vi "HFRR ADV v02.vi"() -> ()   [LabVIEW 2025] (continued)
            n811 = call "CAMERA LIVE FEED FGV.vi"("Enum - Menu"=CAMERA_LIVE_FEED_ENUM."CAMERA MINIMIZE") -> ()  [unwired: 9 in, 2 out]
          }
        }
        n812 = local write "CAMERA ROI MAX TEMP"(TRUE ("CAMERA ROI MAX TEMP")) -> ()
        n813 = case shown="True" w1177 {
          selector: w1177 -> [_ w1183]
          frame False {
          }
          frame True {
            n814 = Not(x=w1183) -> (.not. x?=w1182:bool)
            n815 = local write "CAMERA ROI MIN TEMP"(w1182) -> ()
            n816 = call "IMAGE ANALYSIS.vi"("Enum"=POST_ANALYSIS_ENUM."MINIMIZE UI") -> ()  [unwired: 9 in, 2 out]
          }
        }
      }
    }
    n817 = local read "Auto Start Test"() -> (w928:bool)
    n818 = case shown="True" "sign in temp" {
      frame False {
      }
      frame True {
        w965 = 1 ("y")
        n819 = local read "USERNAME"() -> (w971:string)
        n820 = local read "USER ID"() -> (w968:string)
        n821 = call <vilib>:"Trim Whitespace.vi"("string"=w971) -> ("trimmed string"=w970:string)  [unwired: 1 in]
        n822 = call <vilib>:"Trim Whitespace.vi"("string"=w968) -> ("trimmed string"=w969:string)  [unwired: 1 in]
        n823 = String Length(string=w970) -> (length=w967:i32)
        n824 = String Length(string=w969) -> (length=w966:i32)
        n825 = Greater?(x=w967, y=w965) -> (0:w964:bool)
        n826 = Greater?(x=w966, y=w965) -> (0:w963:bool)
        n827 = And(x=w964, y=w963) -> (x .and. y?=w962:bool)
        n828 = case shown="True" w962 {
          frame False {
            n829 = property on="Sign In" class="Bool (strict)"("DisabledEnum"=T13."Disabled" ("Disabled")) -> ()  [unwired: 2 in, 2 out]
          }
          frame True {
            n830 = property on="Sign In" class="Bool (strict)"("DisabledEnum"=T13."Enabled" ("Disabled")) -> ()  [unwired: 2 in, 2 out]
          }
        }
      }
    }
    n831 = local read "Air Temperature"() -> (w945:bool)
    n832 = local read "Coefficient Of Friction"() -> (w946:bool)
    n833 = case shown="False" w928 {
      frame False {
        n834 = local read "Auto stop temp"() -> (w959:bool)
        n835 = case shown="True" w959 {
          frame False {
          }
          frame True {
            n836 = local write "Auto Start Temp"(FALSE ("Auto Start Temp")) -> ()
          }
        }
      }
      frame True {
        "Auto stop temp" <- TRUE ("Auto stop temp")
      }
    }
    n837 = local read "Humidity"() -> (w944:bool)
    n838 = case shown="\"HOME\"" w956 {
      frame "HOME" {
        n839 = local write "main tab sub"(enum32{"Page 1", "Page 2"}."Page 1" ("main tab sub")) -> ()
      }
      frame Default {
        n840 = local write "main tab sub"(enum32{"Page 1", "Page 2"}."Page 2" ("main tab sub")) -> ()
      }
    }
    n841 = case shown="True" w955 {
      selector: w955 -> [_ w1291]
      frame False {
      }
      frame True {
        n842 = Not(x=w1291) -> (.not. x?=w1290:bool)
        n843 = local write "Sign In"(w1290) -> ()
        n844 = local write "Main Dashboard Buttons"(T1."Test Setup" ("Main Dashboard Buttons")) -> ()
      }
    }
    n845 = case shown="\"Numeric Display\", Default" "Num/Graph" {
      frame "Numeric Display", Default {
        n846 = property on="Single/Multiple" class="RadioBtnsControl (strict)"("Visible"=FALSE) -> ()  [unwired: 2 in, 2 out]
        n847 = property on="Single - Graph" class="Ring (strict)"("Visible"=FALSE) -> ()  [unwired: 2 in, 2 out]
        n848 = local write "Main Tab Display"(T4."Dashboard 1" ("Main Tab Display")) -> ()
      }
      frame "Graph Display" {
        n849 = property on="Single/Multiple" class="RadioBtnsControl (strict)"("Visible"=TRUE) -> ()  [unwired: 2 in, 2 out]
        n850 = case shown="\"Multiple\"" "Single/Multiple" {
          frame "Single ", Default {
            n851 = property on="Single - Graph" class="Ring (strict)"("Visible"=TRUE) -> ()  [unwired: 2 in, 2 out]
            n852 = local write "Main Tab Display"(T4."Dashboard 3" ("Main Tab Display")) -> ()
          }
          frame "Multiple" {
            n853 = property on="Single - Graph" class="Ring (strict)"("Visible"=FALSE) -> ()  [unwired: 2 in, 2 out]
            n854 = local write "Main Tab Display"(T4."Dashboard 2" ("Main Tab Display")) -> ()
          }
        }
      }
    }
    n855 = local read "Stroke"() -> (w943:bool)
    n856 = local read "USERNAME"() -> (w949:string)
    n857 = local read "USER ID"() -> (w948:string)
    n858 = case shown="True" w946 {
      selector: w946 -> [_ w1226]
      frame False {
      }
      frame True {
        n859 = Not(x=w1226) -> (.not. x?=w1225:bool)
        n860 = local write "Coefficient Of Friction"(w1225) -> ()
        n861 = local write "Tab Control 2"(T6."Coefficient Of Friction" ("Tab Control 2")) -> ()
      }
    }
    n862 = case shown="True" w945 {
      selector: w945 -> [_ w1223]
      frame False {
      }
      frame True {
        n863 = Not(x=w1223) -> (.not. x?=w1221:bool)
        n864 = local write "Air Temperature"(w1221) -> ()
        n865 = local write "Tab Control 2"(T6."Air Temperature" ("Tab Control 2")) -> ()
      }
    }
    n866 = local write "Operator ID"(w948) -> ()
    n867 = case shown="True" w943 {
      selector: w943 -> [_ w1217]
      frame False {
      }
      frame True {
        n868 = Not(x=w1217) -> (.not. x?=w1215:bool)
        n869 = local write "Stroke"(w1215) -> ()
        n870 = local write "Tab Control 2"(T6."Stroke" ("Tab Control 2")) -> ()
      }
    }
    n871 = local write "tested by"(w949) -> ()
    n872 = case shown="True" w944 {
      selector: w944 -> [_ w1220]
      frame False {
      }
      frame True {
        n873 = Not(x=w1220) -> (.not. x?=w1218:bool)
        n874 = local write "Humidity"(w1218) -> ()
        n875 = local write "Tab Control 2"(T6."Humidity" ("Tab Control 2")) -> ()
      }
    }
    n876 = case shown="\"Advance\"" "Main Dashboard Buttons" {
      tunnel: [T2."HOME" ("Main Tab") T2."Test Setup" ("Main Tab") T2."Acquire" ("Main Tab") T2."Adv Scar" ("Main Tab") T2."Adv Scar Report" ("Main Tab") T2."Compare Files" ("Main Tab") T2."About" ("Main Tab") T2."Advance" ("Main Tab")] -> w953
      frame "Home", Default {
      }
      frame "Test Setup" {
      }
      frame "Dashboard" {
      }
      frame "Imaging" {
      }
      frame "Report" {
      }
      frame "Analysis" {
      }
      frame "About" {
      }
      frame "Advance" {
      }
    }
    n877 = Wait (ms)(milliseconds to wait=u32 100) -> ()  [unwired: 1 out]
    n878 = local read "Main Tab Display"() -> (w947:T4)
    n879 = local write "Main Tab"(w953) -> ()
    n880 = case shown="\"Dashboard 3\"" w947 {
      frame "Dashboard 1", Default {
        n881 = property on="Reset Graph" class="Bool (strict)"("Visible"=FALSE) -> ()  [unwired: 2 in, 2 out]
      }
      frame "Dashboard 2" {
        n882 = property on="Reset Graph" class="Bool (strict)"("Visible"=TRUE) -> ()  [unwired: 2 in, 2 out]
      }
      frame "Dashboard 3" {
        n883 = property on="Reset Graph" class="Bool (strict)"("Visible"=TRUE) -> ()  [unwired: 2 in, 2 out]
      }
    }
    n884 = local read "SCAR MEASURMENT"() -> (w935:enum32{"Auto Scar", "Manual Scar"})
    n885 = local read "Humidity"() -> (w950:bool)
    n886 = local read "Cap Live Image"() -> (w932:bool)
    n887 = local read "Sample Temperature"() -> (w942:bool)
    n888 = local read "Air Temp vs Humidity"() -> (w940:bool)
    n889 = local read "Frequency"() -> (w941:bool)
    n890 = case shown="False" w950 {
      frame False {
        n891 = local write "Humidity On Command"(TRUE ("Humidity On Command")) -> ()
        n892 = case shown="True" "Humidity Off Command" {
          selector: "Humidity Off Command" -> [_ w1233]
          frame False {
          }
          frame True {
            n893 = stacked-sequence {
              frame #0 {
                n894 = local read "WriteHumidity"() -> (w1235:string[])
                n895 = Insert Into Array(array=w1235, new element="R;1" ("new element/subarray")) -> (w1236:string[])  [unwired: 1 in]
                n896 = local write "WriteHumidity"(w1236) -> ()
              }
              frame #1 {
                n897 = Wait (ms)(milliseconds to wait=u32 2000) -> ()  [unwired: 1 out]
              }
              frame #2 {
                n898 = local read "EVENT LOG"() -> (w1242:string)
                n899 = local read "WriteHumidity"() -> (w1239:string[])
                n900 = call "Event Log.vi"("Content"="Humidity Control Off" ("string"), "EVENT LOG"=w1242) -> ("EVENT LOG"=w1243:string)  [unwired: 8 in, 1 out]
                n901 = local write "EVENT LOG"(w1243) -> ()
                n902 = Insert Into Array(array=w1239, new element="R;1" ("new element/subarray")) -> (w1240:string[])  [unwired: 1 in]
                n903 = local write "WriteHumidity"(w1240) -> ()
              }
            }
            n904 = Not(x=w1233) -> (.not. x?=w1232:bool)
            n905 = local write "Humidity Off Command"(w1232) -> ()
          }
        }
      }
      frame True {
        n906 = local write "Humidity Off Command"(TRUE ("Humidity Off Command")) -> ()
        n907 = case shown="False" "Humidity On Command" {
          selector: "Humidity On Command" -> [_ w1247]
          frame False {
          }
          frame True {
            n908 = stacked-sequence {
              frame #0 {
                n909 = local read "Set Rh"() -> (w1253:dbl)
                n910 = Number To Fractional String(number=w1253, precision (6)=i16 2) -> (F-format string=w1254:string)  [unwired: 2 in]
                n911 = local read "WriteHumidity"() -> (w1251:string[])
                n912 = Concatenate Strings("M;" ("new element/subarray"), w1254) -> (w1252:string)
                n913 = Insert Into Array(array=w1251, new element=w1252) -> (w1250:string[])  [unwired: 1 in]
                n914 = local write "WriteHumidity"(w1250) -> ()
              }
              frame #1 {
                n915 = Wait (ms)(milliseconds to wait=u32 1500) -> ()  [unwired: 1 out]
              }
              frame #2 {
                (unwired) "% RH" ("string")
                (unwired) i16 2 ("precision (6)")
                (unwired) "M;" ("new element/subarray")
                n916 = local read "Set Rh"() -> (w1261:dbl)
                n917 = Number To Fractional String(number=w1261, precision (6)=i16 2) -> (F-format string=w1258:string)  [unwired: 2 in]
                n918 = local read "WriteHumidity"() -> (w1263:string[])
                n919 = Concatenate Strings("M;" ("new element/subarray"), w1258) -> (w1262:string)
                n920 = Concatenate Strings("Humidity Set to : " ("string"), w1258, "% RH" ("string")) -> (w1256:string)
                n921 = Insert Into Array(array=w1263, new element=w1262) -> (w1264:string[])  [unwired: 1 in]
                n922 = disable-structure shown="Enabled" {
                  frame Enabled {
                    n923 = local read "EVENT LOG"() -> (w1267:string)
                    n924 = call "Event Log.vi"("Content"="Humidity Control On", "EVENT LOG"=w1267) -> ("EVENT LOG"=w1268:string)  [unwired: 8 in, 1 out]
                    n925 = local write "EVENT LOG"(w1268) -> ()
                  }
                  frame Disabled {
                  }
                }
                n926 = disable-structure shown="Enabled" {
                  disable-tunnel: w1256 -> [_ _]
                  frame Enabled {
                    n927 = local read "EVENT LOG"() -> (w1270:string)
                    n928 = call "Event Log.vi"("Content"="Humidity Control On", "EVENT LOG"=w1270) -> ("EVENT LOG"=w1271:string)  [unwired: 8 in, 1 out]
                    n929 = local write "EVENT LOG"(w1271) -> ()
                  }
                  frame Disabled {
                  }
                }
                n930 = local write "WriteHumidity"(w1264) -> ()
              }
            }
            n931 = Not(x=w1247) -> (.not. x?=w1246:bool)
            n932 = local write "Humidity On Command"(w1246) -> ()
          }
        }
      }
    }
    n933 = Equal?(x=w935, y=enum32{"Auto Scar", "Manual Scar"}."Auto Scar" ("SCAR MEASURMENT")) -> (x = y?=w931:bool)
    n934 = local read "TEST STANDARD"() -> (w938:T3)
    n935 = And(x=w932, y=w931) -> (x .and. y?=w933:bool)
    n936 = case shown="True" w933 {
      selector: w933 -> [_ w1032]
      tunnel: errorcluster {"status"=FALSE, "code"=0, "source"=""} ("error in (no error) 3") -> [_ w1033]
      frame False {
      }
      frame True {
        n937 = stacked-sequence {
          tunnel: w1033 -> [_ _ _ _ _ _ _ w1081]
          tunnel: w1032 -> [_ _ _ _ _ w1062 _ _]
          frame #0 {
            n938 = call "CAMERA LIVE FEED FGV.vi"("Enum - Menu"=CAMERA_LIVE_FEED_ENUM."CAMERA MINIMIZE") -> ()  [unwired: 9 in, 2 out]
          }
          frame #1 {
            n939 = property on="Auto Scar Check  2" class="Clust (strict)"("Visible"=TRUE) -> ()  [unwired: 2 in, 2 out]
          }
          frame #2 {
            n940 = String To Path(string="C:\\LAB-IQ\\Image Calibrate v01.dcf") -> (path=w1038:path)
            n941 = Open/Create/Replace File ("Open File")(file path (use dialog)=w1038) -> (refnum out=w1039:refnum<file>)  [unwired: 5 in, 2 out]
            n942 = for {
              N: 4 -> [_]
              tunnel: w1039 -> [w1045]
              i -> [w1041]
              n943 = Read from Text File ("Read File")(file (use dialog)=w1045) -> (text=w1046:string)  [unwired: 3 in, 3 out]
              n944 = String Subset(string=w1046, offset (0)=6, length (rest)=10 ("length (rest)")) -> (substring=w1042:string)
              n945 = Fract/Exp String To Number(string=w1042) -> (number=w1040:dbl)  [unwired: 3 in, 1 out]
              n946 = case shown="0" w1041 {
                tunnel: w1040 -> [w1047 w1048 _ w1049 _]
                frame 0 {
                  "5x Gain" <- w1047
                }
                frame 1 {
                  "10x Gain" <- w1048
                }
                frame 2 {
                }
                frame 3 {
                  "100x gain" <- w1049
                }
                frame 4, Default {
                }
              }
            }
          }
          frame #3 {
            n947 = local read "FILE 3"() -> (w1055:string)
            n948 = call <vilib>:"Trim Whitespace.vi"("string"="C:\\LAB-IQ\\images\\") -> ("trimmed string"=w1057:string)  [unwired: 1 in]
            n949 = String To Path(string=w1057) -> (path=w1056:path)
            n950 = Concatenate Strings(w1055, ".png" ("string")) -> (w1054:string)
            n951 = Build Path(base path=w1056, name or relative path=w1054) -> (appended path=w1052:path)
            "Image path" <- w1052
            n952 = Path To String(path=w1052) -> (string=w1051:string)
            n953 = call "CAMERA LIVE FEED FGV.vi"("Enum - Menu"=CAMERA_LIVE_FEED_ENUM."CAMERA SAVE", "Image Path"=w1051) -> ()  [unwired: 8 in, 2 out]
          }
          frame #4 {
            n954 = One Button Dialog(message="Image saved successfully") -> ()  [unwired: 1 in, 1 out]
          }
          frame #5 {
            n955 = local read "TEST STANDARD"() -> (w1061:T3)
            n956 = local read "Magnification len live scar"() -> (w1073:string)
            n957 = Not(x=w1062) -> (.not. x?=w1063:bool)
            n958 = local write "Cap Live Image"(w1063) -> ()
            n959 = case shown="\"ISO 12156\"" w1061 {
              tunnel: ["ASTM D6079" "ISO 12156"] -> w1060
              frame "ASTM D6079", Default {
              }
              frame "ISO 12156" {
              }
            }
            n960 = case shown="\"5x\", Default" w1073 {
              tunnel: [w1076 w1077] -> w1072
              frame "5x", Default {
                n961 = local read "5x Gain"() -> (w1076:dbl)
              }
              frame "10x" {
                # "5x"
                n962 = local read "10x Gain"() -> (w1077:dbl)
              }
            }
            n963 = local read "Image path"() -> (w1071:path)
            n964 = local read "FILE 3"() -> (w1064:string)
            n965 = call "EDGE DETCTION.vi"("GAIN VALUE"=w1072, "Image Path"=w1071) -> ("error out"=w1070:errorcluster, "return value"=w1069:cluster{string, string, dbl, dbl, dbl})  [unwired: 8 in]
            n966 = Bundle By Name(cluster=T18 {"File Name"="", "Test Method"="", "Operator"="", "Fuel Description"="", "Date and time"=""} ("Main Ref"), "File Name"=w1064, "Test Method"=w1060) -> (w1065:T18)
            n967 = call "duf file read.vi"("error in (no error)"=w1070, "Main Ref"=w1065) -> ("error out"=w1068:errorcluster, "Main Ref 2"=w1066:T18)  [unwired: 8 in]
            n968 = call "EDGE DETECTION REPORT.vi"("error in (no error)"=w1068, "return value 2"=w1069, "Main Ref"=w1066) -> ()  [unwired: 8 in, 1 out]
          }
          frame #6 {
            n969 = property on="Auto Scar Check  2" class="Clust (strict)"("Visible"=FALSE) -> ()  [unwired: 2 in, 2 out]
          }
          frame #7 {
            n970 = call "CAMERA LIVE FEED FGV.vi"("Enum - Menu"=CAMERA_LIVE_FEED_ENUM."CAMERA MINIMIZE", "error in (no error)"=w1081) -> ()  [unwired: 8 in, 2 out]
            n971 = local write "Main Dashboard Buttons"(T1."Home" ("Main Dashboard Buttons")) -> ()
            n972 = local write "Main Tab"(T2."HOME" ("Main Tab")) -> ()
          }
        }
      }
    }
    n973 = local read "Heater Button"() -> (w939:bool)
    n974 = case shown="True" w941 {
      selector: w941 -> [_ w1211]
      frame False {
      }
      frame True {
        n975 = Not(x=w1211) -> (.not. x?=w1209:bool)
        n976 = local write "Frequency"(w1209) -> ()
        n977 = local write "Tab Control 2"(T6."Frequency" ("Tab Control 2")) -> ()
      }
    }
    n978 = case shown="True" w940 {
      selector: w940 -> [_ w1208]
      frame False {
      }
      frame True {
        n979 = Not(x=w1208) -> (.not. x?=w1206:bool)
        n980 = local write "Air Temp vs Humidity"(w1206) -> ()
        n981 = local write "Tab Control 2"(T6."Air Temp vs Rh" ("Tab Control 2")) -> ()
      }
    }
    n982 = case shown="True" w942 {
      selector: w942 -> [_ w1214]
      frame False {
      }
      frame True {
        n983 = Not(x=w1214) -> (.not. x?=w1212:bool)
        n984 = local write "Sample Temperature"(w1212) -> ()
        n985 = local write "Tab Control 2"(T6."Sample Temperature" ("Tab Control 2")) -> ()
      }
    }
    n986 = case shown="\"Custom\"" w938 {
      frame "ASTM D6079", Default {
        w1187 = "ASTM D6079 TEST CONDITIONS" ("Standard 2")
        n987 = local write "Standard 2"(w1187) -> ()
        n988 = local write "Standard"(w1187) -> ()
      }
      frame "ISO 12156" {
        w1188 = "ISO 12156 TEST CONDITIONS" ("Standard 2")
        n989 = local write "Standard 2"(w1188) -> ()
        n990 = local write "Standard"(w1188) -> ()
      }
      frame "CEC F-096-A-06" {
        w1189 = "CEC F-096-A-06 TEST CONDITIONS" ("Standard 2")
        n991 = local write "Standard 2"(w1189) -> ()
        n992 = local write "Standard"(w1189) -> ()
      }
      frame "Custom" {
        w1190 = "CUSTOM TEST CONDITIONS" ("Standard 2")
        n993 = local write "Standard 2"(w1190) -> ()
        n994 = local write "Standard"(w1190) -> ()
      }
    }
    n995 = case shown="True" w939 {
      frame False {
        n996 = local write "Temperature On Command"(TRUE ("Temperature On Command")) -> ()
        n997 = case shown="True" "Temperature Off Command" {
          selector: "Temperature Off Command" -> [_ w1194]
          frame False {
          }
          frame True {
            n998 = Not(x=w1194) -> (.not. x?=w1193:bool)
            n999 = local read "EVENT LOG"() -> (w1197:string)
            n1000 = local write "Temperature Off Command"(w1193) -> ()
            n1001 = call "Event Log.vi"("Content"="Heater Off", "EVENT LOG"=w1197) -> ("EVENT LOG"=w1196:string)  [unwired: 8 in, 1 out]
            n1002 = local write "EVENT LOG"(w1196) -> ()
          }
        }
      }
      frame True {
        n1003 = local write "Temperature Off Command"(TRUE ("Temperature Off Command")) -> ()
        n1004 = case shown="True" "Temperature On Command" {
          selector: "Temperature On Command" -> [_ w1201]
          frame False {
          }
          frame True {
            n1005 = Not(x=w1201) -> (.not. x?=w1200:bool)
            n1006 = local write "Temperature On Command"(w1200) -> ()
            n1007 = disable-structure shown="Enabled" {
              disable-tunnel: "Heater On" -> [w1203 _]
              frame Enabled {
                n1008 = local read "EVENT LOG"() -> (w1204:string)
                n1009 = call "Event Log.vi"("Content"=w1203, "EVENT LOG"=w1204) -> ("EVENT LOG"=w1205:string)  [unwired: 8 in, 1 out]
                n1010 = local write "EVENT LOG"(w1205) -> ()
              }
              frame Disabled {
              }
            }
          }
        }
      }
    }
    n1011 = local read "Main Tab"() -> (w930:T2)
    n1012 = case shown="\"About\"" w930 {
      frame "HOME", Default {
        w976 = T13."Enabled" ("Disabled")
        n1013 = local read "Service Password enable"() -> (w975:bool)
        n1014 = property on="Imaging" class="Bool (strict)"("DisabledEnum"=w976) -> ()  [unwired: 2 in, 2 out]
        n1015 = property on="Dashboard" class="Bool (strict)"("DisabledEnum"=w976) -> ()  [unwired: 2 in, 2 out]
        n1016 = property on="Test Setup" class="Bool (strict)"("DisabledEnum"=w976) -> ()  [unwired: 2 in, 2 out]
        n1017 = property on="Analysis" class="Bool (strict)"("DisabledEnum"=w976) -> ()  [unwired: 2 in, 2 out]
        n1018 = property on="Home" class="Bool (strict)"("DisabledEnum"=w976) -> ()  [unwired: 2 in, 2 out]
        n1019 = property on="Report" class="Bool (strict)"("DisabledEnum"=w976) -> ()  [unwired: 2 in, 2 out]
        n1020 = property on="Main Dashboard Buttons" class="RadioBtnsControl (strict)"("DisabledEnum"=w976) -> ()  [unwired: 2 in, 2 out]
        n1021 = case shown="True" w975 {
          tunnel: [T13."Disabled" ("Disabled") T13."Enabled" ("Disabled")] -> w974
          frame False {
          }
          frame True {
          }
        }
        n1022 = property on="About" class="Bool (strict)"("DisabledEnum"=w974) -> ()  [unwired: 2 in, 2 out]
      }
      frame "Test Setup" {
        w981 = T13."Enabled" ("Disabled")
        n1023 = local read "Service Password enable"() -> (w980:bool)
        n1024 = property on="Dashboard" class="Bool (strict)"("DisabledEnum"=T13."Disabled" ("Disabled")) -> ()  [unwired: 2 in, 2 out]
        n1025 = property on="Imaging" class="Bool (strict)"("DisabledEnum"=w981) -> ()  [unwired: 2 in, 2 out]
        n1026 = property on="Analysis" class="Bool (strict)"("DisabledEnum"=w981) -> ()  [unwired: 2 in, 2 out]
        n1027 = property on="Home" class="Bool (strict)"("DisabledEnum"=w981) -> ()  [unwired: 2 in, 2 out]
        n1028 = property on="Report" class="Bool (strict)"("DisabledEnum"=w981) -> ()  [unwired: 2 in, 2 out]
        n1029 = property on="Test Setup" class="Bool (strict)"("DisabledEnum"=w981) -> ()  [unwired: 2 in, 2 out]
        n1030 = case shown="True" w980 {
          tunnel: [T13."Disabled" ("Disabled") T13."Enabled" ("Disabled")] -> w979
          frame False {
          }
          frame True {
          }
        }
        n1031 = property on="About" class="Bool (strict)"("DisabledEnum"=w979) -> ()  [unwired: 2 in, 2 out]
      }
      frame "Adv Scar" {
        w988 = T13."Enabled" ("Disabled")
        n1032 = property on="Dashboard" class="Bool (strict)"("DisabledEnum"=T13."Disabled" ("Disabled")) -> ()  [unwired: 2 in, 2 out]
        n1033 = property on="Imaging" class="Bool (strict)"("DisabledEnum"=w988) -> ()  [unwired: 2 in, 2 out]
        n1034 = property on="Analysis" class="Bool (strict)"("DisabledEnum"=w988) -> ()  [unwired: 2 in, 2 out]
        n1035 = property on="Home" class="Bool (strict)"("DisabledEnum"=w988) -> ()  [unwired: 2 in, 2 out]
        n1036 = property on="Report" class="Bool (strict)"("DisabledEnum"=w988) -> ()  [unwired: 2 in, 2 out]
        n1037 = property on="Test Setup" class="Bool (strict)"("DisabledEnum"=w988) -> ()  [unwired: 2 in, 2 out]
        n1038 = local read "Service Password enable"() -> (w986:bool)
        n1039 = case shown="True" w986 {
          tunnel: [T13."Disabled" ("Disabled") T13."Enabled" ("Disabled")] -> w985
          frame False {
          }
          frame True {
          }
        }
        n1040 = property on="About" class="Bool (strict)"("DisabledEnum"=w985) -> ()  [unwired: 2 in, 2 out]
      }
      frame "Adv Scar Report" {
        w993 = T13."Enabled" ("Disabled")
        n1041 = property on="Dashboard" class="Bool (strict)"("DisabledEnum"=T13."Disabled" ("Disabled")) -> ()  [unwired: 2 in, 2 out]
        n1042 = property on="Imaging" class="Bool (strict)"("DisabledEnum"=w993) -> ()  [unwired: 2 in, 2 out]
        n1043 = property on="Analysis" class="Bool (strict)"("DisabledEnum"=w993) -> ()  [unwired: 2 in, 2 out]
        n1044 = property on="Home" class="Bool (strict)"("DisabledEnum"=w993) -> ()  [unwired: 2 in, 2 out]
        n1045 = property on="Report" class="Bool (strict)"("DisabledEnum"=w993) -> ()  [unwired: 2 in, 2 out]
        n1046 = property on="Test Setup" class="Bool (strict)"("DisabledEnum"=w993) -> ()  [unwired: 2 in, 2 out]
        n1047 = local read "Service Password enable"() -> (w992:bool)
        n1048 = case shown="True" w992 {
          tunnel: [T13."Disabled" ("Disabled") T13."Enabled" ("Disabled")] -> w991
          frame False {
          }
          frame True {
          }
        }
        n1049 = property on="About" class="Bool (strict)"("DisabledEnum"=w991) -> ()  [unwired: 2 in, 2 out]
      }
      frame "Compare Files" {
        w999 = T13."Enabled" ("Disabled")
        n1050 = local read "Service Password enable"() -> (w998:bool)
        n1051 = property on="Dashboard" class="Bool (strict)"("DisabledEnum"=T13."Disabled" ("Disabled")) -> ()  [unwired: 2 in, 2 out]
        n1052 = property on="Imaging" class="Bool (strict)"("DisabledEnum"=w999) -> ()  [unwired: 2 in, 2 out]
        n1053 = property on="Analysis" class="Bool (strict)"("DisabledEnum"=w999) -> ()  [unwired: 2 in, 2 out]
        n1054 = property on="Home" class="Bool (strict)"("DisabledEnum"=w999) -> ()  [unwired: 2 in, 2 out]
        n1055 = property on="Report" class="Bool (strict)"("DisabledEnum"=w999) -> ()  [unwired: 2 in, 2 out]
        n1056 = property on="Test Setup" class="Bool (strict)"("DisabledEnum"=w999) -> ()  [unwired: 2 in, 2 out]
        n1057 = case shown="True" w998 {
          tunnel: [T13."Disabled" ("Disabled") T13."Enabled" ("Disabled")] -> w997
          frame False {
          }
          frame True {
          }
        }
        n1058 = property on="About" class="Bool (strict)"("DisabledEnum"=w997) -> ()  [unwired: 2 in, 2 out]
      }
      frame "Acquire" {
        n1059 = local read "Service Password enable"() -> (w1003:bool)
        n1060 = property on="Test Setup" class="Bool (strict)"("DisabledEnum"=T13."Disabled" ("Disabled")) -> ()  [unwired: 2 in, 2 out]
        n1061 = local read "Auto Start Test"() -> (w1005:bool)
        n1062 = local read "RUN"() -> (w1007:bool)
        n1063 = case shown="True" w1003 {
          tunnel: [T13."Disabled" ("Disabled") T13."Enabled" ("Disabled")] -> w1004
          frame False {
          }
          frame True {
          }
        }
        n1064 = Or(x=w1007, y=w1005) -> (x .or. y?=w1006:bool)
        n1065 = case shown="True" w1006 {
          tunnel: [T13."Enabled" ("Disabled") T13."Disabled" ("Disabled")] -> w1009
          frame False {
          }
          frame True {
          }
        }
        n1066 = property on="About" class="Bool (strict)"("DisabledEnum"=w1004) -> ()  [unwired: 2 in, 2 out]
        n1067 = property on="Imaging" class="Bool (strict)"("DisabledEnum"=w1009) -> ()  [unwired: 2 in, 2 out]
        n1068 = property on="Dashboard" class="Bool (strict)"("DisabledEnum"=w1009) -> ()  [unwired: 2 in, 2 out]
        n1069 = property on="Analysis" class="Bool (strict)"("DisabledEnum"=w1009) -> ()  [unwired: 2 in, 2 out]
        n1070 = property on="Home" class="Bool (strict)"("DisabledEnum"=w1009) -> ()  [unwired: 2 in, 2 out]
        n1071 = property on="Report" class="Bool (strict)"("DisabledEnum"=w1009) -> ()  [unwired: 2 in, 2 out]
      }
      frame "About" {
        n1072 = local read "FILE"() -> (w1022:string)
        n1073 = local read "TEST FILE NAM,E SAVED"() -> (w1015:bool)
        n1074 = call <vilib>:"Trim Whitespace.vi"("string"=w1022) -> ("trimmed string"=w1021:string)  [unwired: 1 in]
        n1075 = local read "Auto Start Test"() -> (w1025:bool)
        n1076 = String Length(string=w1021) -> (length=w1020:i32)
        n1077 = Greater?(x=w1020, y=1) -> (0:w1017:bool)
        n1078 = And(x=w1017, y=w1015) -> (x .and. y?=w1016:bool)
        n1079 = local read "RUN"() -> (w1027:bool)
        n1080 = case shown="True" w1016 {
          tunnel: [T13."Disabled" ("Disabled") T13."Enabled" ("Disabled")] -> w1018
          frame False {
          }
          frame True {
          }
        }
        n1081 = Or(x=w1027, y=w1025) -> (x .or. y?=w1026:bool)
        n1082 = property on="About" class="Bool (strict)"("DisabledEnum"=T13."Enabled" ("Disabled")) -> ()  [unwired: 2 in, 2 out]
        n1083 = case shown="False" w1026 {
          tunnel: [T13."Enabled" ("Disabled") T13."Disabled" ("Disabled")] -> w1024
          frame False {
          }
          frame True {
          }
        }
        n1084 = property on="Dashboard" class="Bool (strict)"("DisabledEnum"=w1018) -> ()  [unwired: 2 in, 2 out]
        n1085 = property on="Test Setup" class="Bool (strict)"("DisabledEnum"=T13."Disabled" ("Disabled")) -> ()  [unwired: 2 in, 2 out]
        n1086 = property on="Imaging" class="Bool (strict)"("DisabledEnum"=w1024) -> ()  [unwired: 2 in, 2 out]
        n1087 = property on="Analysis" class="Bool (strict)"("DisabledEnum"=w1024) -> ()  [unwired: 2 in, 2 out]
        n1088 = property on="Home" class="Bool (strict)"("DisabledEnum"=w1024) -> ()  [unwired: 2 in, 2 out]
        n1089 = property on="Report" class="Bool (strict)"("DisabledEnum"=w1024) -> ()  [unwired: 2 in, 2 out]
      }
    }
    n1090 = local read "Quit"() -> (w958:bool)
    "Single" <- "Single - Graph"
  }
  n1091 = disable-structure shown="Disabled" {
    disable-tunnel: [w1295 _] -> w39
    disable-tunnel: _ -> [w1294 _]
    frame Disabled {
      n1092 = while {
        tunnel: w1294 -> [_]
        tunnel: [w1296] -> w1295
        tunnel: [w1297] -> _
        i -> [w1297]
        stop <- w1296 stop-if-true
        w1313 = u16 10 items=["1.0"=10, "1.5"=15, "2.0"=20] ("stop bits (10: 1 bit)")
        n1093 = Wait (ms)(milliseconds to wait=u32 10) -> ()  [unwired: 1 out]
        n1094 = call-poly "VISA Configure Serial Port"("VISA resource name"=refnum<visa-resource-name> "ASRL1::INSTR" ("COM PORT"), "timeout (10sec)"=u32 10, "baud rate (9600)"=u32 57600, "data bits (8)"=u16 8, "stop bits (10: 1 bit)"=w1313) -> ("VISA resource name out"=w1299:refnum<visa-resource-name>, "error out"=w1308:errorcluster)  [unwired: 9 in]
        n1095 = VISA Read(VISA resource name=w1299, byte count=u32 2 ("byte count (0)")) -> (read buffer=w1307:string)  [unwired: 1 in, 3 out]
        n1096 = String Subset(string=w1307, offset (0)=0, length (rest)=2 ("length (rest)")) -> (substring=w1306:string)
        n1097 = Match Pattern(string=w1306, regular expression="<>") -> (offset past match=w1303:i32)  [unwired: 1 in, 3 out]
        n1098 = Greater Or Equal?(x=w1303, y=0) -> (x >= y?=w1298:bool)
        n1099 = case shown="True" w1298 {
          tunnel: w1299 -> [_ w1317]
          tunnel: w1308 -> [_ w1316]
          frame False {
          }
          frame True {
            n1100 = VISA Read(VISA resource name=w1317, byte count=u32 32 ("byte count (0)"), error in (no error)=w1316) -> (read buffer=w1315:string)  [unwired: 3 out]
            n1101 = String Subset(string=w1315, offset (0)=0, length (rest)=8 ("length (rest)")) -> (substring=w1319:string)
            n1102 = String Subset(string=w1315, offset (0)=8, length (rest)=8 ("length (rest)")) -> (substring=w1320:string)
            n1103 = Decimal String To Number(string=w1320) -> (number=w1327:i32)  [unwired: 2 in, 1 out]
            n1104 = Decimal String To Number(string=w1319) -> (number=w1323:i32)  [unwired: 2 in, 1 out]
            n1105 = Divide(x=w1327, y=10000) -> ()  [unwired: 1 out]
            n1106 = Divide(x=w1323, y=1000000) -> ()  [unwired: 1 out]
          }
        }
        n1107 = local read "Quit"() -> (w1296:bool)
      }
    }
    frame Enabled {
    }
  }
  n1108 = while {
    shift-right: [w1342] -> w52
    shift-left: _ -> [w1333]
    shift-right: [w1341] -> w51
    shift-left: errorcluster {"status"=TRUE, "code"=0, "source"="Init"} ("error IO") -> [w1335]
    tunnel: [w1330] -> w42
    tunnel: [w1340] -> _
    i -> [w1340]
    stop <- w1330 stop-if-true
    n1109 = local read "Port 1a"() -> (w1336:bool)
    n1110 = local read "Port 3"() -> (w1337:bool)
    n1111 = local read "Com Port 1"() -> (w1334:refnum<visa-resource-name>)
    n1112 = Or(x=w1337, y=w1336) -> (x .or. y?=w1339:bool)
    n1113 = Unbundle(w1335) -> ("status"=→"Port 3":bool)  [unwired: 2 out]
    n1114 = Not Equal?(x=w1334, y=w1333) -> (x != y?=w1331:bool)
    n1115 = case shown="True" w1339 {
      frame False {
        w1345 = FALSE ("Visible")
        n1116 = property on="Port 1a" class="Bool (strict)"("Visible"=w1345) -> ()  [unwired: 2 in, 2 out]
        n1117 = property on="Port 3" class="Bool (strict)"("Visible"=w1345) -> ()  [unwired: 2 in, 2 out]
      }
      frame True {
        w1346 = TRUE ("Visible")
        n1118 = property on="Port 1a" class="Bool (strict)"("Visible"=w1346) -> ()  [unwired: 2 in, 2 out]
        n1119 = property on="Port 3" class="Bool (strict)"("Visible"=w1346) -> ()  [unwired: 2 in, 2 out]
      }
    }
    n1120 = Wait (ms)(milliseconds to wait=u32 10) -> ()  [unwired: 1 out]
    n1121 = case shown="True" w1331 {
      tunnel: [w1343 errorcluster {"status"=TRUE, "code"=0, "source"="Init"} ("error out")] -> w1332
      tunnel: w1335 -> [w1343 _]
      frame False {
      }
      frame True {
      }
    }
    n1122 = case shown="No Error" w1332 {
      selector: w1332 -> [w1353 w1380]
      tunnel: [w1356 w1384] -> w1342
      tunnel: [w1355 w1378] -> w1341
      tunnel: w1333 -> [w1354 w1382]
      frame No Error {
        n1123 = property class="Instr"(reference=w1354, error in=w1353) -> (reference out=w1351:refnum<visa-resource-name>, error out=w1352:errorcluster, "Serial Settings:Number of Bytes at Serial Port"=w1347:u32)
        n1124 = Greater?(x=w1347, y=u32 5) -> (0:w1349:bool)
        n1125 = Not(x=w1349) -> (.not. x?=→"Port 1a":bool)
        n1126 = while {
          tunnel: [w1373] -> w1355
          tunnel: [w1372] -> w1356
          tunnel: w1352 -> [w1371]
          tunnel: w1351 -> [w1370]
          stop <- TRUE stop-if-true
          n1127 = property class="Instr" props=["Serial Settings:Number of Bytes at Serial Port"](reference=w1370, error in=w1371) -> (reference out=w1375:refnum<visa-resource-name>, error out=w1374:errorcluster)  [unwired: 1 out]
          n1128 = VISA Read(VISA resource name=w1375, byte count=u32 1000, error in (no error)=w1374) -> (VISA resource name out=w1372:refnum<visa-resource-name>, read buffer=w1357:string, error out=w1373:errorcluster)  [unwired: 1 out]
          "UNI READ" <- w1357
          n1129 = Spreadsheet String To Array(delimiter (Tab)=";", format string="", spreadsheet string=w1357, array type (2D Dbl)=dbl[] []) -> (array=w1367:dbl[])
          n1130 = Index Array(array=w1367) -> (element #1=→"LVDT MIN":dbl, element #2=→"LVDT MAX":dbl, element #3=→"LVDT Peak":dbl, element #4=→"pizo raw":dbl, element #5=→"Friction":dbl, element #6=→"cof 2":dbl)  [unwired: 6 in]
        }
      }
      frame Error {
        w1390 = u16 0 items=["None", "XON/XOFF", "RTS/CTS", "XON/XOFF & RTS/CTS", "DTR/DSR", "XON/XOFF & DTR/DSR"] ("flow control (0:none)  2")
        w1388 = u16 10 items=["1.0"=10, "1.5"=15, "2.0"=20] ("stop bits 2")
        w1386 = u16 0 items=["None", "Odd", "Even", "Mark", "Space"] ("parity 2")
        w1387 = u32 10000  # timeout (10sec)
        n1131 = VISA Close(VISA resource name=w1382, error in (no error)=w1380) -> (error out=w1383:errorcluster)
        n1132 = local write "Port 1a"(FALSE ("Port 1a")) -> ()
        n1133 = local read "Com Port 1"() -> (w1377:refnum<visa-resource-name>)
        n1134 = call <vilib>:"Clear Errors.vi"("error in (no error)"=w1383) -> ("error out"=w1381:errorcluster)  [unwired: 5 in, 1 out]
        n1135 = call-poly "VISA Configure Serial Port"("VISA resource name"=w1377, "timeout (10sec)"=w1387, "baud rate (9600)"=u32 250000 ("baud rate  2"), "data bits (8)"=u16 8 ("data bits  2"), "parity (0:none)"=w1386, "error in (no error)"=w1381, "stop bits (10: 1 bit)"=w1388, "flow control (0:none)"=w1390) -> ("VISA resource name out"=w1391:refnum<visa-resource-name>, "error out"=w1392:errorcluster)  [unwired: 6 in]
        n1136 = flat-sequence {
          tunnel: w1391 -> [w1394]
          tunnel: w1392 -> [w1393]
          tunnel: [w1394] -> w1384
          tunnel: [w1393] -> w1378
          frame #0 {
            n1137 = Wait (ms)(milliseconds to wait=u32 50) -> ()  [unwired: 1 out]
          }
        }
        "Residual Uno" <- ""
        "Port 1 Error" <- w1378
      }
    }
    n1138 = local read "Quit"() -> (w1330:bool)
    "Error Uno" <- w1335
  }
  n1139 = while {
    stop <- w1401 stop-if-true
    # "V0OLTAGE TO STROKE (peice vise calibration)"
    n1140 = Wait (ms)(milliseconds to wait=u32 10) -> ()  [unwired: 1 out]
    n1141 = local read "LVDT Peak"() -> (w1398:dbl)
    n1142 = formula code="// Dynamic Parameterized Linear Interpolation Node\n// Inputs: vpp_val, voltages (Array), distances (Array)\n// Outputs: stroke\n\nint i = 0;\nint segments = 11; // 12 points make 11 interpolation segments\n\n// 1. Lower Boundary Clamp\nif (vpp_val <= voltages[0]) {\n    stroke = distances[0];\n}\n// 2. Upper Boundary Clamp\nelse if (vpp_val >= voltages[segments]) {\n    stroke = distances[segments];\n}\n// 3. Dynamic Segment Search Loop\nelse {\n    stroke = distances[0]; // Fallback baseline\n    for (i = 0; i < segments; i++) {\n        if (vpp_val >= voltages[i] && vpp_val <= voltages[i+1]) {\n            // Standard linear interpolation formula using array lookups\n            stroke = distances[i] + (vpp_val - voltages[i]) * (distances[i+1] - distances[i]) / (voltages[i+1] - voltages[i]);\n            break; // Segment found, safely exit the loop\n        }\n    }\n}"("vpp_val"=w1398, "voltages"="calibration values", "distances"="STROKE") -> ("stroke"=w1397:dbl)
    n1143 = local write "measured_stroke"(w1397) -> ()
    n1144 = local read "Quit"() -> (w1401:bool)
  }
  n1145 = while {
    shift-right: [w1415] -> w37
    shift-left: _ -> [w1406]
    shift-right: [w1414] -> w36
    shift-left: errorcluster {"status"=FALSE, "code"=0, "source"="Init"} ("error out") -> [w1408]
    tunnel: [w1403] -> w41
    tunnel: [w1413] -> _
    i -> [w1413]
    stop <- w1403 stop-if-true
    n1146 = local read "Com Port 2"() -> (w1407:refnum<visa-resource-name>)
    n1147 = local read "Port 2a"() -> (w1409:bool)
    n1148 = Unbundle(w1408) -> ("status"=→"Port 4":bool)  [unwired: 2 out]
    n1149 = call <vilib>:"High Resolution Polling Wait.vi"("seconds to wait"=0.2) -> ()  [unwired: 10 in, 1 out]
    n1150 = local read "Port 4"() -> (w1410:bool)
    n1151 = Not Equal?(x=w1407, y=w1406) -> (x != y?=w1405:bool)
    n1152 = Or(x=w1410, y=w1409) -> (x .or. y?=w1412:bool)
    n1153 = case shown="True" w1412 {
      frame False {
        w1418 = FALSE ("Visible")
        n1154 = property on="Port 2a" class="Bool (strict)"("Visible"=w1418) -> ()  [unwired: 2 in, 2 out]
        n1155 = property on="Port 4" class="Bool (strict)"("Visible"=w1418) -> ()  [unwired: 2 in, 2 out]
      }
      frame True {
        w1419 = TRUE ("Visible")
        n1156 = property on="Port 2a" class="Bool (strict)"("Visible"=w1419) -> ()  [unwired: 2 in, 2 out]
        n1157 = property on="Port 4" class="Bool (strict)"("Visible"=w1419) -> ()  [unwired: 2 in, 2 out]
      }
    }
    n1158 = case shown="True" w1405 {
      tunnel: [w1416 errorcluster {"status"=TRUE, "code"=0, "source"="Init"} ("error out")] -> w1404
      tunnel: w1408 -> [w1416 _]
      frame False {
      }
      frame True {
      }
    }
    n1159 = case shown="No Error" w1404 {
      selector: w1404 -> [w1435 w1466]
      tunnel: [w1422 w1471] -> w1415
      tunnel: [w1436 w1464] -> w1414
      tunnel: w1406 -> [w1438 w1469]
      frame No Error {
        n1160 = property class="Instr"(reference=w1438, error in=w1435) -> (reference out=w1429:refnum<visa-resource-name>, error out=w1434:errorcluster, "Serial Settings:Number of Bytes at Serial Port"=w1425:u32)
        n1161 = while {
          tunnel: [w1446] -> w1430
          tunnel: [w1445] -> w1431
          tunnel: w1434 -> [w1444]
          tunnel: w1429 -> [w1443]
          tunnel: [w1442] -> _
          i -> [w1442]
          stop <- TRUE stop-if-true
          n1162 = property class="Instr" props=["Serial Settings:Number of Bytes at Serial Port"](reference=w1443, error in=w1444) -> (reference out=w1448:refnum<visa-resource-name>, error out=w1447:errorcluster)  [unwired: 1 out]
          n1163 = VISA Read(VISA resource name=w1448, byte count=u32 1000, error in (no error)=w1447) -> (VISA resource name out=w1445:refnum<visa-resource-name>, read buffer=→"Due read":string, error out=w1446:errorcluster)  [unwired: 1 out]
        }
        n1164 = Greater?(x=w1425, y=u32 23) -> (0:w1427:bool)
        n1165 = Not(x=w1427) -> ()  [unwired: 1 out]
        n1166 = call "Elapsed Time10"("Time Target (s)"=2.0, "Reset"=w1427, "Auto Reset"=FALSE) -> ("Time has Elapsed"=→"Port 2a":bool)  [unwired: 9 in, 7 out]
        n1167 = local read "Command"() -> (w1420:string)
        n1168 = Not Equal?(x=w1420, y="") -> (x != y?=w1432:bool)
        n1169 = case shown="True" w1432 {
          tunnel: w1431 -> [w1450 w1456]
          tunnel: [w1450 w1460] -> w1437
          tunnel: w1430 -> [w1449 w1455]
          tunnel: [w1449 w1458] -> w1436
          tunnel: w1420 -> [_ w1454]
          tunnel: [_ w1457] -> _
          frame False {
            # "DATA  WRITE LOOP"
          }
          frame True {
            n1170 = Concatenate Strings(w1454, "\r\n") -> (w1453:string)
            n1171 = VISA Write(VISA resource name=w1456, write buffer=w1453, error in (no error)=w1455) -> (VISA resource name out=w1460:refnum<visa-resource-name>, return count=w1457:u32, error out=w1459:errorcluster)
            n1172 = flat-sequence {
              tunnel: w1459 -> [w1461]
              tunnel: [w1461] -> w1458
              frame #0 {
                n1173 = Wait (ms)(milliseconds to wait=u32 5) -> ()  [unwired: 1 out]
              }
            }
            n1174 = local write "Command"("" ("Command")) -> ()
          }
        }
        n1175 = VISA Flush I/O Buffer(VISA resource name=w1437) -> (VISA resource name out=w1422:refnum<visa-resource-name>, error out=→"error out 9":errorcluster)  [unwired: 2 in]
      }
      frame Error {
        w1477 = u16 0 items=["None", "XON/XOFF", "RTS/CTS", "XON/XOFF & RTS/CTS", "DTR/DSR", "XON/XOFF & DTR/DSR"] ("flow control (0:none)  2")
        w1475 = u16 10 items=["1.0"=10, "1.5"=15, "2.0"=20] ("stop bits 2")
        w1473 = u16 0 items=["None", "Odd", "Even", "Mark", "Space"] ("parity 2")
        w1474 = u32 10000  # timeout (10sec)
        n1176 = VISA Clear(VISA resource name=w1469, error in (no error)=w1466) -> (VISA resource name out=w1468:refnum<visa-resource-name>, error out=w1467:errorcluster)
        n1177 = VISA Close(VISA resource name=w1468, error in (no error)=w1467) -> (error out=w1470:errorcluster)
        n1178 = call <vilib>:"Clear Errors.vi"("error in (no error)"=w1470) -> ()  [unwired: 5 in, 2 out]
        n1179 = local read "Com Port 2"() -> (w1463:refnum<visa-resource-name>)
        "visa due" <- w1463
        n1180 = call-poly "VISA Configure Serial Port"("VISA resource name"=w1463, "timeout (10sec)"=w1474, "baud rate (9600)"=u32 250000 ("baud rate  2"), "data bits (8)"=u16 8 ("data bits  2"), "parity (0:none)"=w1473, "stop bits (10: 1 bit)"=w1475, "flow control (0:none)"=w1477) -> ("VISA resource name out"=w1478:refnum<visa-resource-name>, "error out"=w1479:errorcluster)  [unwired: 7 in]
        n1181 = flat-sequence {
          tunnel: w1478 -> [w1481]
          tunnel: w1479 -> [w1480]
          tunnel: [w1481] -> w1471
          tunnel: [w1480] -> w1464
          frame #0 {
            n1182 = Wait (ms)(milliseconds to wait=u32 50) -> ()  [unwired: 1 out]
          }
        }
        "Residual Due" <- ""
        "Port 2 Error" <- w1464
      }
    }
    n1183 = local read "Quit"() -> (w1403:bool)
    "Error Due" <- w1408
  }
  n1184 = local write "FRICVALZ"(0.0 ("FRICVALZ")) -> ()
  n1185 = property on="RUN" class="Bool (strict)"("Visible"=TRUE) -> ()  [unwired: 2 in, 2 out]
  n1186 = while {
    tunnel: [w1498] -> _
    tunnel: [w1483] -> w54
    i -> [w1498]
    stop <- w1483 stop-if-true
    n1187 = local read "conststatus"() -> (w1487:dbl)
    n1188 = local read "Main Tab"() -> (w1485:T2)
    n1189 = local read "EDIT"() -> (w1504:bool)
    n1190 = local read "Rate"() -> (w1503:dbl)
    n1191 = case shown="True" w1504 {
      tunnel: [FALSE TRUE] -> w1490
      frame False {
      }
      frame True {
      }
    }
    n1192 = property on="Time slide" class="Slide (strict)"("Scale.Range:Maximum"=2500.0) -> ()  [unwired: 2 in, 2 out]
    n1193 = Equal?(x=w1485, y=T20."About" ("Main Tab")) -> (x = y?=w1496:bool)
    n1194 = Equal?(x=w1487, y=0.0) -> (x = y?=w1488:bool)
    n1195 = Divide(x=1.0, y=w1503) -> (x/y=w1499:dbl)
    "Time 2" <- w1499
    n1196 = case shown="True" w1488 {
      frame False {
      }
      frame True {
        # "C:\\WinDucom\\calibrate WO 2391.dcf"
        n1197 = local write "Lan flag"(22) -> ()
        n1198 = local write "conststatus"(10.0 ("rpm value : 2")) -> ()
        n1199 = String To Path(string="C:\\LAB-IQ\\calibrate WO 2465.dcf") -> (path=w1510:path)
        n1200 = Open/Create/Replace File "Open File"(file path (use dialog)=w1510) -> (refnum out=w1508:refnum<file>)  [unwired: 5 in, 2 out]
        n1201 = for {
          N: 23 -> [_]
          tunnel: w1508 -> [w1519]
          i -> [w1513]
          (unwired) TRUE ("line mode (F)")
          n1202 = Read from Text File "Read File"(file (use dialog)=w1519) -> (text=w1518:string)  [unwired: 3 in, 3 out]
          n1203 = Match Pattern(string=w1518, regular expression="]") -> (after substring=w1516:string)  [unwired: 1 in, 3 out]
          n1204 = String Subset(string=w1518, offset (0)=5, length (rest)=10 ("length (rest)")) -> (substring=w1511:string)
          n1205 = Fract/Exp String To Number(string=w1511) -> (number=w1512:dbl)  [unwired: 3 in, 1 out]
          n1206 = Match Pattern(string=w1516, regular expression="-") -> (before substring=w1514:string)  [unwired: 1 in, 3 out]
          n1207 = case shown="5" w1513 {
            tunnel: w1512 -> [w1522 w1523 w1524 w1525 _ _ _ w1530 w1531 _ w1532 w1533 w1534 w1535 w1536 w1537 _ w1538 w1539 _ _ _ _ _]
            tunnel: w1514 -> [_ _ _ _ w1526 w1527 w1528 _ _ _ _ _ _ _ _ _ _ _ _ w1540 w1541 _ w1542 _]
            frame 0 {
              n1208 = local write "FRIC. FORCE :"(w1522) -> ()
            }
            frame 1 {
              n1209 = local write "TEMPERATURE :"(w1523) -> ()
            }
            frame 2 {
              n1210 = local write "HUMIDITY:"(w1524) -> ()
            }
            frame 3 {
              n1211 = local write "AIR TEMPERATURE :"(w1525) -> ()
            }
            frame 4 {
              n1212 = local write "Com Port 1"(w1526) -> ()
            }
            frame 5 {
              n1213 = local write "Com Port 2"(w1527) -> ()
              n1214 = local write "visa due"(w1527) -> ()
            }
            frame 6 {
              n1215 = String To Path(string=w1528) -> (path=w1529:path)
              n1216 = local write "File Path"(w1529) -> ()
              "String" <- w1528
            }
            frame 7 {
              n1217 = local write "DISPLACEMENT :"(w1530) -> ()
            }
            frame 8 {
              n1218 = local write "STROKE GAIN :"(w1531) -> ()
            }
            frame 9 {
            }
            frame 10 {
              n1219 = local write "Language Selection"(w1532) -> ()
            }
            frame 11 {
              n1220 = local write "CH-POWER +"(w1533) -> ()
            }
            frame 12 {
              n1221 = local write "CH-POWER -"(w1534) -> ()
            }
            frame 13 {
              n1222 = local write "CH-HEATER"(w1535) -> ()
            }
            frame 14 {
              n1223 = local write "CH-HUMIDITY WET"(w1536) -> ()
            }
            frame 15 {
              n1224 = local write "CH-HUMIDITY DRY"(w1537) -> ()
            }
            frame 16 {
            }
            frame 17 {
              n1225 = local write "AIR TEMP INTERCEPT:"(w1538) -> ()
            }
            frame 18 {
              n1226 = local write "TEMP INTERCEPT:"(w1539) -> ()
            }
            frame 19 {
              n1227 = local write "S.NO"(w1540) -> ()
            }
            frame 20 {
              n1228 = local write "Com Port 3"(w1541) -> ()
            }
            frame 21 {
            }
            frame 22 {
              n1229 = local write "C3 :"(w1542) -> ()
            }
            frame 23, Default {
            }
          }
        }
      }
    }
    n1230 = Select(t=u32 2500 ("milliseconds to wait"), s=w1496, f=u32 500 ("milliseconds to wait")) -> (s? t:f=w1494:u32)
    n1231 = Multiply(x=w1499, y=w1494) -> (x*y=w1501:dbl)
    n1232 = property on="Time slide" class="Slide (strict)"("Visible"=w1490) -> ()  [unwired: 2 in, 2 out]
    n1233 = call "Elapsed Time2"("Time Target (s)"=w1501, "Auto Reset"=TRUE) -> ("Time has Elapsed"=w1491:bool)  [unwired: 10 in, 7 out]
    n1234 = case shown="True" w1491 {
      frame False {
      }
      frame True {
        n1235 = stacked-sequence {
          frame #0 {
            w1543 = 0.0
            # "DATA PROCESSING"
            # "115 mV/N"
            n1236 = local read "RH Numeric:"() -> (w1549:dbl)
            n1237 = local read "HUMIDITY:"() -> (w1550:dbl)
            n1238 = local read "FRICVALZ"() -> (w1561:dbl)
            n1239 = local read "Friction"() -> (w1544:dbl)
            n1240 = local write "TEMP"(w1543) -> ()
            n1241 = Multiply(x=w1549, y=w1550) -> (x*y=→"Humidity ( %RH )" →"Hum" →"Hum 2":dbl)
            n1242 = Subtract(x=w1544, y=w1561) -> (x-y=w1556:dbl)
            "FF 2" <- w1556
            "FF 4" <- w1556
            n1243 = local read "TEMP"() -> (w1560:dbl)
            n1244 = local write "FF 3"(w1556) -> ()
            n1245 = Compound Arithmetic op=OR("FRICVALZ 4", "FRICVALZ 3", "FRICVALZ 2") -> (w1552:bool)
            n1246 = case shown="True" w1552 {
              tunnel: w1544 -> [_ w1567]
              frame False {
              }
              frame True {
                w1566 = FALSE ("FRICVALZ")
                n1247 = local write "FRICVALZ 3"(w1566) -> ()
                n1248 = local write "FRICVALZ 2"(w1566) -> ()
                n1249 = local write "FRICVALZ 4"(w1566) -> ()
                "FRICVALZ" <- w1567
              }
            }
            n1250 = Not A Number/Path/Refnum?(number/path/refnum=w1560) -> (NaN/Path/Refnum?=w1559:bool)
            n1251 = Not A Number/Path/Refnum?(number/path/refnum=w1556) -> (NaN/Path/Refnum?=w1558:bool)
            n1252 = Divide(x=w1556, y=1.96) -> (x/y=w1553:dbl)
            n1253 = Compound Arithmetic op=OR(w1559, w1558) -> (w1557:bool)
            n1254 = Not A Number/Path/Refnum?(number/path/refnum=w1553) -> (NaN/Path/Refnum?=w1554:bool)
            n1255 = case shown="True" w1557 {
              frame False {
              }
              frame True {
                n1256 = local write "TEMP"(0.0 ("TEMP")) -> ()
                n1257 = local write "FF 2"(0.0 ("FF 2")) -> ()
                n1258 = local write "reinit"(TRUE ("reinit")) -> ()
              }
            }
            n1259 = Select(t=0.0, s=w1554, f=w1553) -> (s? t:f=→"COF 2":dbl)
            "AIR TEMP" <- w1543
            "TEMP 2" <- w1543
            "TEMP 3" <- w1543
          }
        }
      }
    }
    n1260 = Wait (ms)(milliseconds to wait=u32 50) -> ()  [unwired: 1 out]
    n1261 = local read "Quit"() -> (w1483:bool)
    "Rate" <- 2500.0 ("No of Samples")
  }
  n1262 = while {
    tunnel: w57 -> [_]
    tunnel: [w1594] -> _
    tunnel: [w1570] -> w56
    i -> [w1594]
    stop <- w1570 stop-if-true
    # "C:\\LAB-IQ-NXT\\Scar View.exe"
    n1263 = local read "OK Button 16"() -> (w1583:bool)
    n1264 = local read "Main Tab"() -> (w1576:T2)
    n1265 = local read "service 3"() -> (w1577:bool)
    n1266 = local read "OPEN 6"() -> (w1579:bool)
    n1267 = local read "EDIT 2"() -> (w1581:bool)
    n1268 = flat-sequence {
      frame #0 {
        n1269 = local read "SAVE 2"() -> (w2196:bool)
        n1270 = stacked-sequence {
          frame #0 {
            n1271 = local read "EDIT"() -> (w2250:bool)
            n1272 = case shown="True" w2250 {
              tunnel: [u8 2 ("Disabled") u8 0 ("Disabled")] -> _
              frame False {
                w2252 = FALSE
                n1273 = local write "Password"("") -> ()
                n1274 = property on="SrvM CP" class="Bool (strict)"("Visible"=w2252) -> ()  [unwired: 2 in, 2 out]
                n1275 = property on="message" class="Str"("Visible"=w2252) -> ()  [unwired: 2 in, 2 out]
                n1276 = local write "x = y?"(w2252) -> ()
                n1277 = property on="Password" class="Str"("Visible"=w2252) -> ()  [unwired: 2 in, 2 out]
                n1278 = property on="ENTER THE NEW PASSWORD" class="Str"("Visible"=w2252) -> ()  [unwired: 2 in, 2 out]
                n1279 = property on="ENTER CURRENT PASSWORD" class="Str"("Visible"=w2252) -> ()  [unwired: 2 in, 2 out]
                n1280 = local write "SrvM CP"(w2252) -> ()
              }
              frame True {
                w2255 = TRUE
                n1281 = property on="SrvM CP" class="Bool (strict)"("Visible"=w2255) -> ()  [unwired: 2 in, 2 out]
                n1282 = property on="Password" class="Str"("Visible"=w2255) -> ()  [unwired: 2 in, 2 out]
              }
            }
            "dipl pwd" <- "@143$\n" ("dipl pwd")
          }
          frame #1 {
            # "Gain password"
            n1283 = String To Byte Array(string="ENTER CURRENT PASSWORD") -> (unsigned byte array=w2260:u8[])
            n1284 = Search 1D Array(1D array=w2260, element=u8 10) -> (index of element=w2263:i32)  [unwired: 1 in]
            n1285 = Index Array(array=w2260, index=w2263) -> (element=w2259:u8)
            n1286 = Equal?(x=w2259, y=10) -> (x = y?=w2257:bool)
            n1287 = case shown="True" w2257 {
              frame False {
                n1288 = property on="ENTER THE NEW PASSWORD" class="Str"("Visible"=FALSE) -> ()  [unwired: 2 in, 2 out]
              }
              frame True {
                # "password"
                # "change password logic"
                n1289 = local read "ENTER CURRENT PASSWORD"() -> (w2276:string)
                n1290 = local read "dipl pwd"() -> (w2270:string)
                n1291 = String To Byte Array(string=w2276) -> (unsigned byte array=w2278:u8[])
                n1292 = String To Byte Array(string=w2270) -> (unsigned byte array=w2271:u8[])
                n1293 = Array Size(array=w2278) -> (size(s)=w2275:i32)
                n1294 = Array Size(array=w2271) -> (size(s)=w2273:i32)
                n1295 = for {
                  N: w2275 -> [_]
                  tunnel: w2278 -> [w2302]
                  tunnel: [w2300] -> w2279 mode=indexing
                  tunnel: w2275 -> [w2294]
                  i -> [w2295]
                  n1296 = Decrement(x=w2294) -> (x-1=w2292:i32)
